vi "EdgeDetector.vi"(1 "Button":bool) -> (0 "Pressed vs Released":bool)   [LabVIEW 2011]
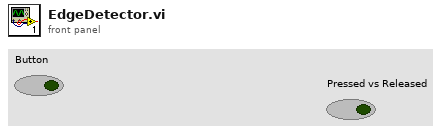
[diagram p1: front panel]
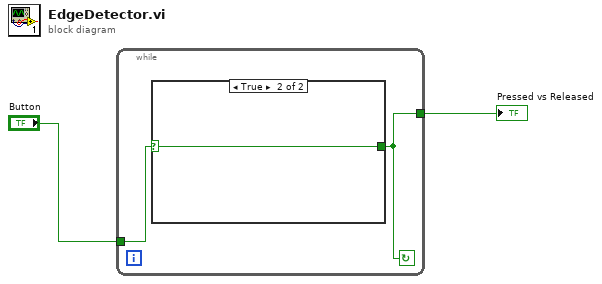
[diagram p0: block diagram]
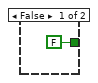
[diagram p2: hidden frame]
diagram:
  n1 = while {
    tunnel: "Button" -> [w4]
    tunnel: [w3] -> w1
    stop <- w3 continue-if-true
    n2 = case shown="True" w4 {
      selector: w4 -> [_ w6]
      tunnel: [FALSE w6] -> w3
      frame False {
      }
      frame True {
      }
    }
  }
  "Pressed vs Released" <- w1
